vi "Close Notifiers.vi"(8 "error in (no error)":errorcluster, 11 "Cluster":T1) -> (0 "error out":errorcluster)   [LabVIEW 2015]
uses:
  Notifiers.ctl
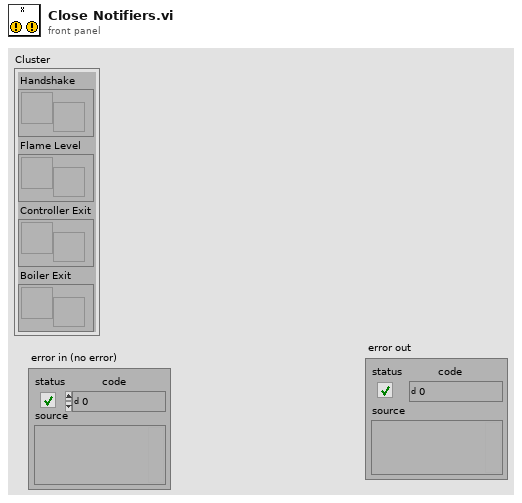
[diagram p1: front panel]
types:
  T1 = typedef "Notifiers.ctl" = cluster{"Handshake":refnum<notifier>, "Flame Level":refnum<notifier>, "Controller Exit":refnum<notifier>, "Boiler Exit":refnum<notifier>}
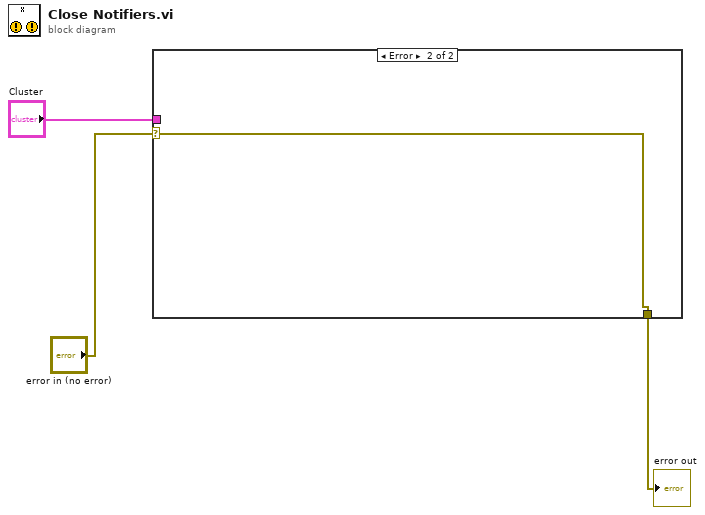
[diagram p0: block diagram]
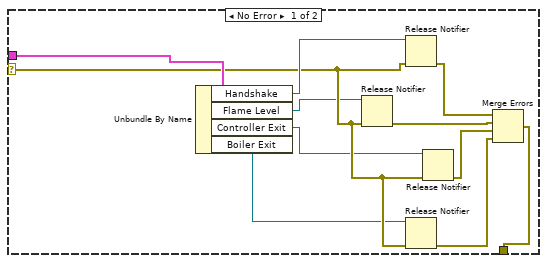
[diagram p2: hidden frame]
diagram:
  n1 = case shown="Error" "error in (no error)" {
    selector: "error in (no error)" -> [w7 w15]
    tunnel: "Cluster" -> [w14 _]
    tunnel: [w9 w15] -> w1
    frame No Error {
      n2 = Unbundle By Name(w14) -> ("Handshake"=w8:refnum<notifier>, "Flame Level"=w6:refnum<notifier>, "Controller Exit"=w5:refnum<notifier>, "Boiler Exit"=w4:refnum<notifier>)
      n3 = Release Notifier(notifier=w6, error in (no error)=w7) -> (error out=w12:errorcluster)  [unwired: 1 in, 2 out]
      n4 = Release Notifier(notifier=w8, error in (no error)=w7) -> (error out=w13:errorcluster)  [unwired: 1 in, 2 out]
      n5 = Release Notifier(notifier=w4, error in (no error)=w7) -> (error out=w10:errorcluster)  [unwired: 1 in, 2 out]
      n6 = Release Notifier(notifier=w5, error in (no error)=w7) -> (error out=w11:errorcluster)  [unwired: 1 in, 2 out]
      n7 = Merge Errors(w13, w12, w11, w10) -> (w9:errorcluster)
    }
    frame Error {
    }
  }
  "error out" <- w1
